vi "clearpath_subscribe.vi"(0 "ClearpathComm":T1, 1 "Frequency":u16, 2 "Message Type":u16(ring)=16384 items=["Echo"=16384, "Platform Info"=16385, "Platform Name"=16386, "Firmware Info"=16387, "System Status"=16388, "Power Status"=16389, "Safety System"=16400, "Differential Speed"=16896, "Differential Control"=16897, "Differential Output"=16898, "Max Speed"=16912, "Max Accel"=16913, "Encoder"=18432, "Raw Encoder"=18433]) -> ()   [LabVIEW 2012, in "clearpath_interface.lvlib"]
doc: "Formats a subscription request given a message type and frequency according to the Clearpath Control Protocol"
uses:
  clearpath_interface.lvlib
  cwrap_crio.dll
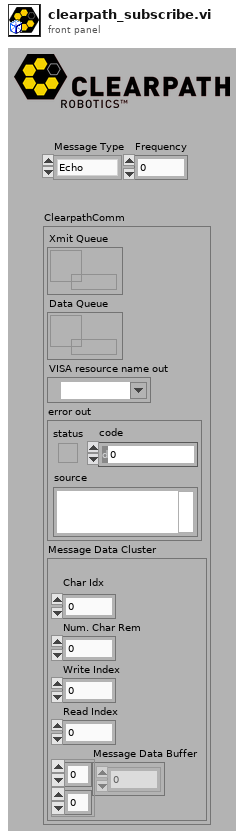
[diagram p1: front panel]
types:
  T1 = cluster{"Xmit Queue":refnum<queue>, "Data Queue":refnum<queue>, "VISA resource name out":refnum<visa-resource-name>, "error out":errorcluster, "Message Data Cluster":cluster{"\nChar Idx":u8, "Num. Char Rem":u8, "Write Index":u8, "Read Index":u8, "Message Data Buffer":u8[][]}}
  T2 = cluster{"buf":u8[], "return type":i32, "Message Type":u16}
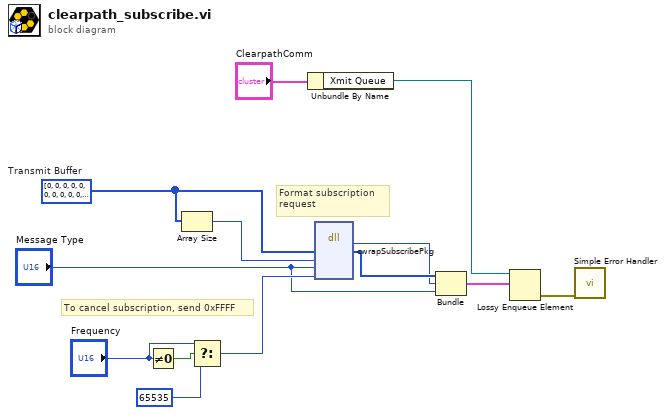
[diagram p0: block diagram]
diagram:
  w12 = u8[] [0, 0, 0, 0, 0, 0, 0, 0, 0, 0, 0, 0, 0, 0, 0, 0, 0, 0, 0, 0, 0, 0, 0, 0, 0, 0, 0, 0, 0, 0, 1, 0, 0, 0, 5]  # Transmit Buffer
  # "Format subscription \nrequest"
  # "To cancel subscription, send 0xFFFF"
  n1 = Not Equal To 0?(x="Frequency") -> (x != 0?=w6:bool)
  n2 = Array Size(array=w12) -> (size(s)=w13:i32)
  n3 = Select(t="Frequency", s=w6, f=u16 65535) -> (s? t:f=w5:u16)
  n4 = Unbundle By Name("ClearpathComm") -> ("Xmit Queue"=w1:refnum<queue>)
  n5 = dll-call lib="C:/Users/whitemrj/Documents/GitHub/IGVC-2013/Code/Project 1.0/Motors/Husky/cwrap_cRIO.*" fn="cwrapSubscribePkg"("buf"=w12, "buf_size"=w13, "type"="Message Type", "freq"=w5) -> ("return type"=w10:i32, "buf"=w11:u8[])  [unwired: 6 in, 2 out]
  n6 = Bundle("buf"=w11, "return type"=w10, "Message Type"="Message Type") -> (w8:T2)  [unwired: 1 in]
  n7 = Lossy Enqueue Element(queue=w1, element=w8) -> (error out=w9:errorcluster)  [unwired: 1 in, 3 out]
  n8 = call <vilib>:"Simple Error Handler.vi"("error in (no error)"=w9) -> ()  [unwired: 4 in, 5 out]
